vi "set State Update User Event.vi"(10 "State Update":T1, 11 "Actor in":refnum<class "Actor.lvclass">) -> (3 "Actor out":refnum<class "Actor.lvclass">)   [LabVIEW 2015, in "Actor.lvclass"]
uses:
  Actor.lvclass
  Update User Event.ctl
  Actor.lvclass/Actor.ctl
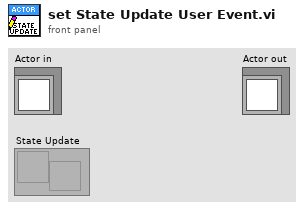
[diagram p1: front panel]
types:
  T1 = typedef "Actor.lvclass/Update User Event.ctl" = refnum<user-event>
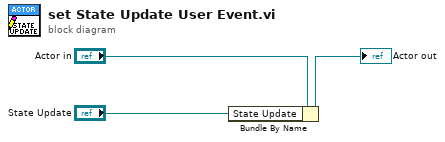
[diagram p0: block diagram]
diagram:
  n1 = Bundle By Name(cluster="Actor in", "State Update"="State Update") -> (→"Actor out":refnum<class "Actor.lvclass">)
